vi "Drawing Tool.vi"() -> ()   [LabVIEW 2020]
doc: "An drawing tool that demonstrates the usage of LabVIEW object oriented programming"
uses:
  Picture/Picture.lvclass
  Graphics Object/Graphics Object.lvclass
  Color/Color.lvclass
  Line/Line.lvclass
  D:/Git/Labview-Libraries/Tools/Drawing Tool Folder/Graphics Object/Graphics Object.lvclass
  Rectangle/Rectangle.lvclass
  Circle/Circle.lvclass
  Triangle/Triangle.lvclass
  Ellipse/Ellipse.lvclass
  Empty/Empty.lvclass
  CMY Color/CMY Color.lvclass
  D:/Git/Labview-Libraries/Tools/Drawing Tool Folder/Color/Color.lvclass
  RGB Color/RGB Color.lvclass
  <vilib>/Utility/cursorutil.llb/Set Cursor (Icon Pict).vi
panel:
  in  "Undo":bool
  out "Colorbox":u32(colorbox)
  in  "Color":enum32{"RGB", "CMY"}(tab)
  in  "Blue RGB":u8(slide) caption="Blue" scale=0.0..255.0
  in  "Green RGB":u8(slide) caption="Green" scale=0.0..255.0
  in  "Red RGB":u8(slide) caption="Red" scale=0.0..255.0
  in  "Yellow CMY":u8(slide)=255 caption="Yellow" scale=0.0..255.0
  in  "Magenta CMY":u8(slide)=255 caption="Magenta" scale=0.0..255.0
  in  "Cyan CMY":u8(slide)=255 caption="Cyan" scale=0.0..255.0
  out "Tools":T1
  out "Picture":picture
  # "Color"
  # "expressionflow"
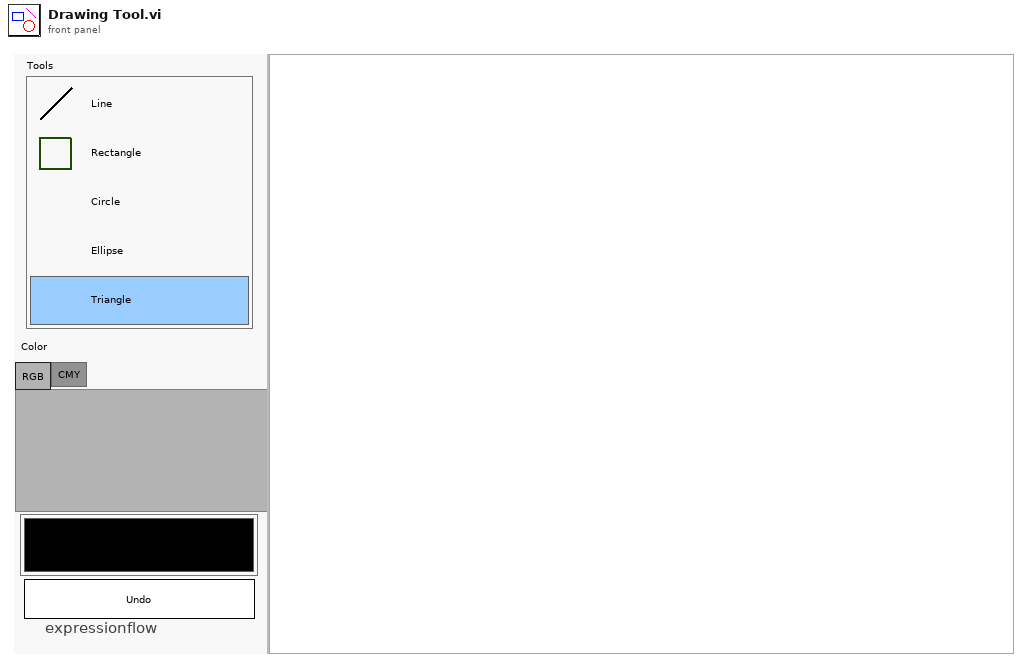
[diagram p1: front panel]
types:
  T1 = cluster{"Line":bool, "Rectangle":bool, "Circle":bool, "Ellipse":bool, "Triangle":bool}
  T2 = cluster{"Picture":refnum<class "Picture.lvclass">, "Tool":refnum<class "Graphics Object.lvclass">, "Unfinished Obj":refnum<class "Graphics Object.lvclass">, "Color":refnum<class "Color.lvclass">, "Tool":refnum<vi>, "Draw mode":bool}
  T3 = typedef "lveventtype.ctl" = enum32{"Null", "Timeout", "Annotation Menu Selection", "Annotation Menu Selection?", "App Instance Close", "App Instance Close?", "Autoscale Range Change", "Bookmark Info Change", "Cell Edit", "Cell Edit?", "Cursor Grab", "Cursor Grab?", "Cursor Menu Selection", "Cursor Menu Selection?", "Cursor Move", "Cursor Release", "Data Change", "Direction Change", "Display State Change", "Drag Ended", "Drag Enter", "Drag Leave", "Drag Over", "Drag Source Update", "Drag Starting", "Drag Starting?", "Drop", "Exec State Change", "Key Down", "Key Down?", "Key Repeat", "Key Repeat?", "Key Up", "Listbox Double Click", "Menu Activation?", "Menu Selection (App)", "Menu Selection? (App)", "Menu Selection (User)", "Mouse Down", "Mouse Down?", "Mouse Enter", "Mouse Leave", "Mouse Move", "Mouse Up", "Mouse Wheel", "NI Security User Change (App)", "Pane Size", "Panel Close", "Panel Close?", "Panel Resize", "Plot Attribute Change", "Scale Range Change", "Shortcut Menu Activation?", "Shortcut Menu Selection (App)", "Shortcut Menu Selection? (App)", "Shortcut Menu Selection (User)", "Tree Double Click", "Tree Drag", "Tree Drag?", "Tree Drop", "Tree Drop?", "Tree Item Close", "Tree Item Close?", "Tree Item Open", "Tree Item Open?", "User Event", "Value Change"}
  T4 = typedef "LVPoint32TypeDef.ctl" = cluster{"Horizontal":i32, "Vertical":i32}
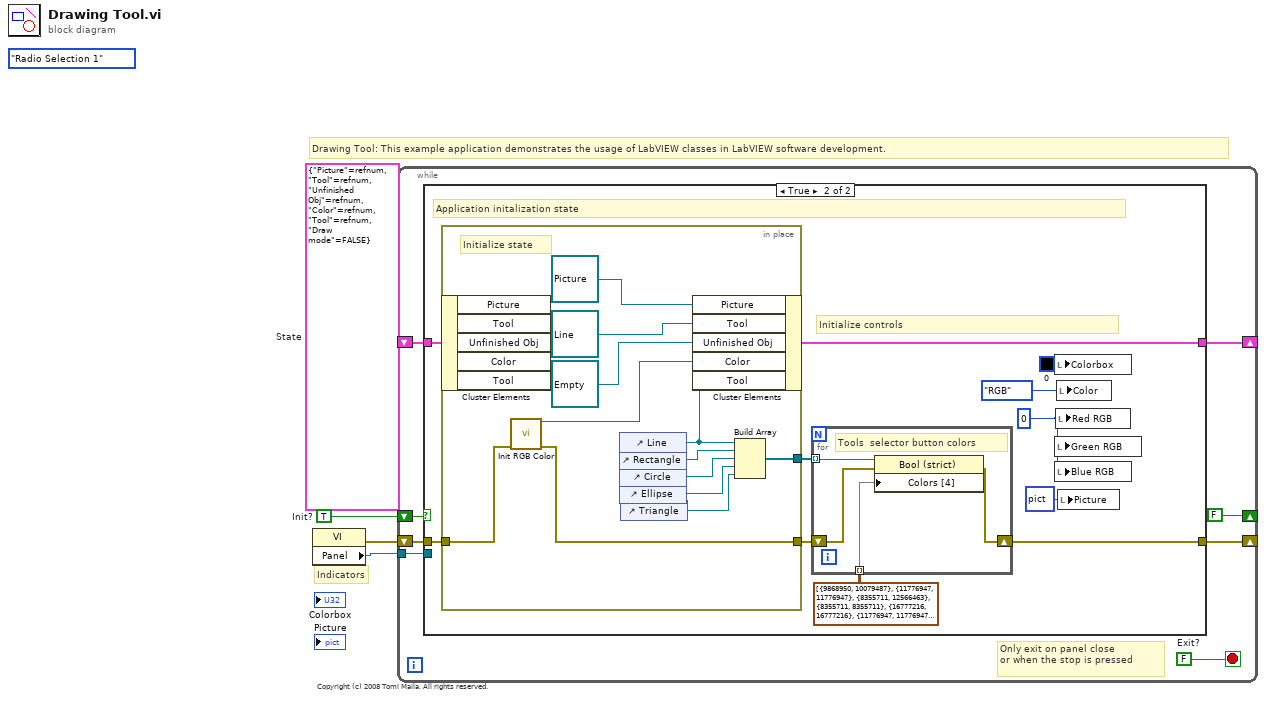
[diagram p0: block diagram]
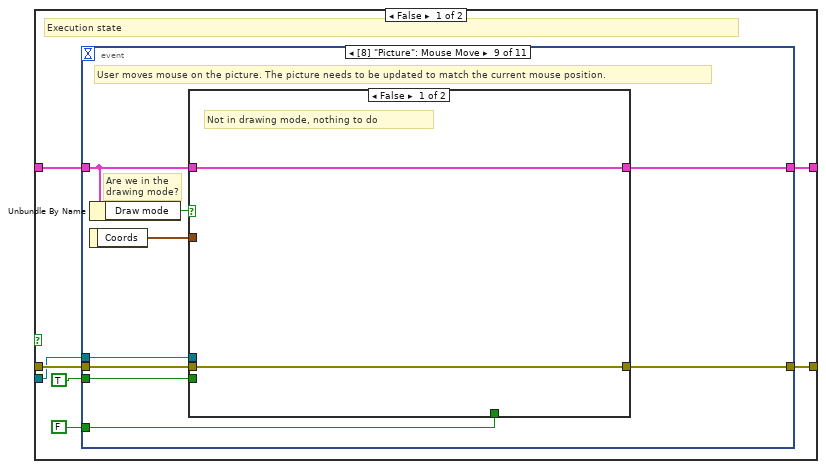
[diagram p2: hidden frame]
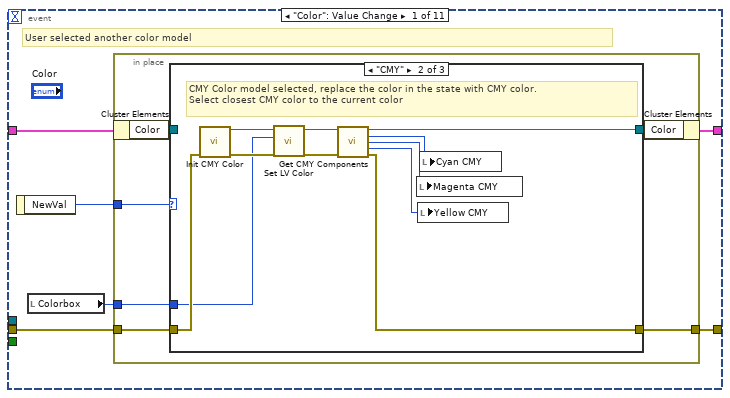
[diagram p3: hidden frame]
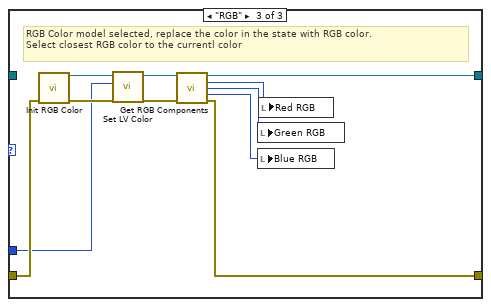
[diagram p5: hidden frame]
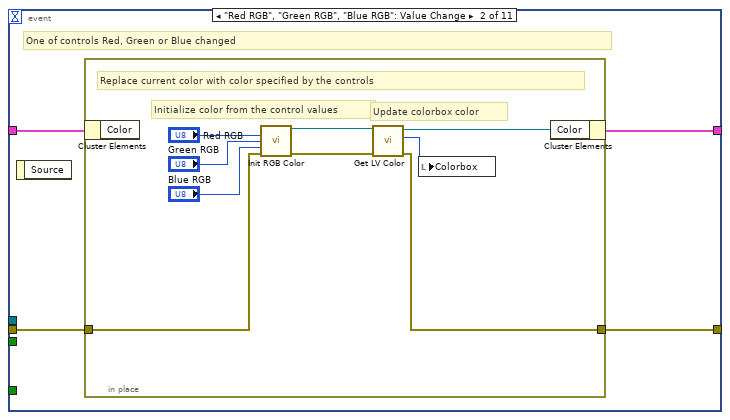
[diagram p6: hidden frame]
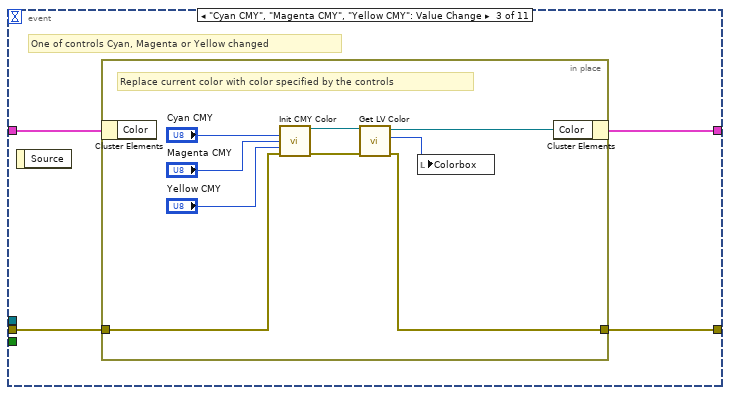
[diagram p7: hidden frame]
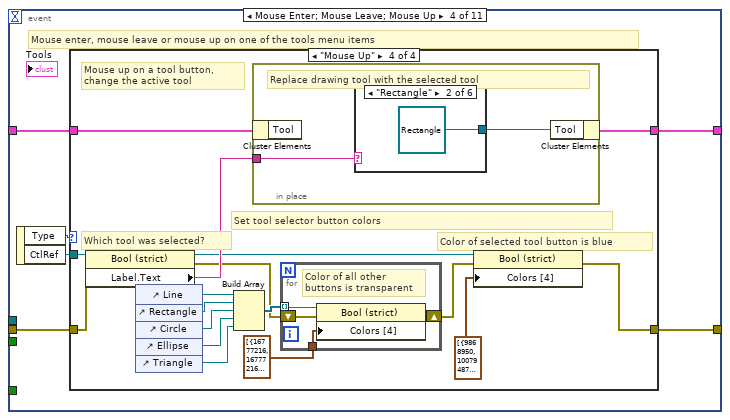
[diagram p8: hidden frame]
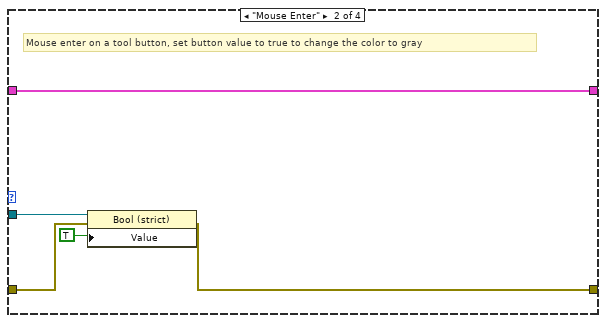
[diagram p10: hidden frame]
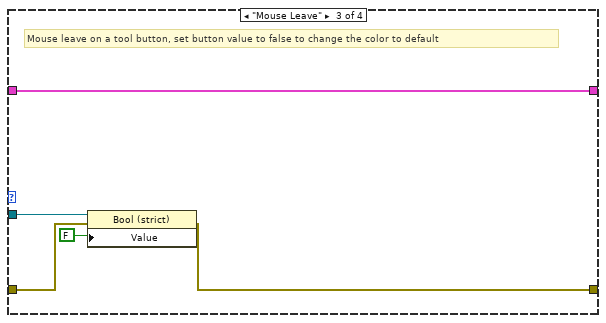
[diagram p11: hidden frame]
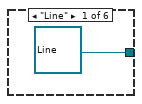
[diagram p12: hidden frame]
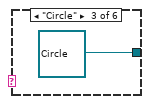
[diagram p13: hidden frame]
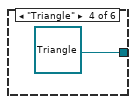
[diagram p14: hidden frame]
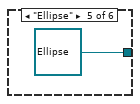
[diagram p15: hidden frame]
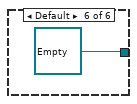
[diagram p16: hidden frame]
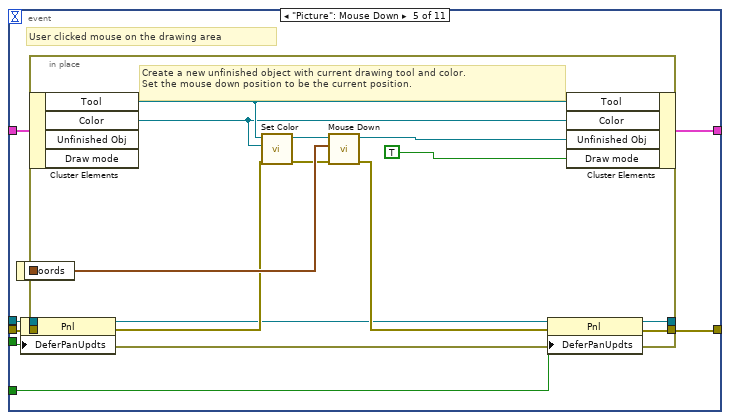
[diagram p17: hidden frame]
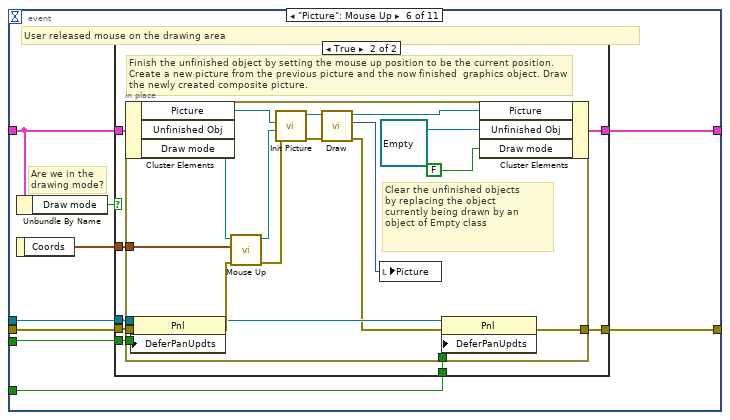
[diagram p18: hidden frame]
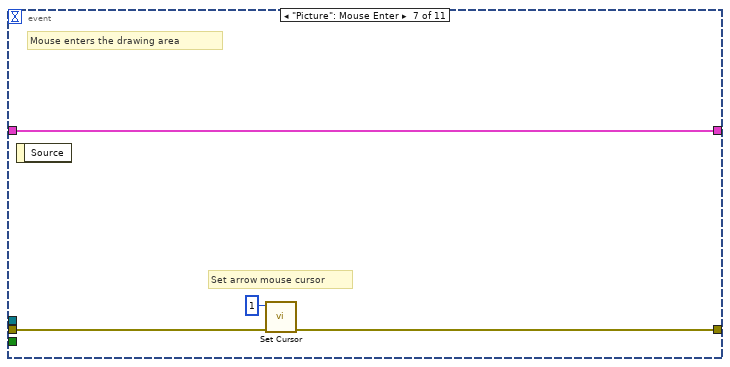
[diagram p20: hidden frame]
diagram:
  w1 = TRUE  # Init?
  w4 = T2 {"Picture"=refnum, "Tool"=refnum, "Unfinished Obj"=refnum, "Color"=refnum, "Tool"=refnum, "Draw mode"=FALSE}  # State
  (unwired) enum32{"Radio Selection 1", "Radio Selection 2"}."Radio Selection 1" ("Radio Buttons")
  # "Copyright (c) 2008 Tomi Maila. All rights reserved."
  # "Drawing Tool: This example application demonstrates the usage of LabVIEW classes in LabVIEW software development."
  # "Indicators"
  n1 = property class="VI"() -> (error out=w2:errorcluster, "Panel"=w3:refnum<vi>)  [unwired: 2 in, 1 out]
  n2 = while {
    shift-right: [w9] -> _
    shift-left: w2 -> [w10]
    shift-right: [w11] -> _
    shift-left: w4 -> [w12]
    tunnel: w3 -> [w7]
    shift-right: [FALSE ("Init?")] -> _
    shift-left: w1 -> [w8]
    stop <- w5 stop-if-true
    w5 = FALSE  # Exit?
    # "Only exit on panel close \nor when the stop is pressed"
    n3 = case shown="True" w8 {
      tunnel: w12 -> [w19 w274]
      tunnel: [w18 w272] -> w11
      tunnel: w10 -> [w17 w273]
      tunnel: w7 -> [w16 _]
      tunnel: [w13 w264] -> w9
      frame False {
        # "Execution state"
        n4 = event shown="[8] \"Picture\": Mouse Move" {
          selector: _ -> [_ _ _ _ _ _ _ _ _ _ _]
          dyn-events: _ -> [_ _ _ _ _ _ _ _ _ _ _]
          timeout: _ -> [_ _ _ _ _ _ _ _ _ _ _]
          tunnel: w17 -> [w25 w59 w72 w85 w134 w154 w191 w196 w205 w245 w259]
          tunnel: [w23 w58 w71 w84 w130 w152 w190 w195 w203 w241 w257] -> w13
          tunnel: w19 -> [w22 w57 w70 w83 w139 w157 w189 w194 w201 w248 w263]
          tunnel: [w21 w56 w69 w82 w138 w159 w189 w193 w207 w247 w263] -> w18
          tunnel: w16 -> [_ _ _ _ w137 w155 _ _ w206 w246 w258]
          tunnel: TRUE -> [_ _ _ _ w133 w153 _ _ w204 w244 _]
          tunnel: FALSE -> [_ _ _ _ w132 w151 _ _ w202 w239 _]
          event "Color": Value Change {
            # "User selected another color model"
            n5 = event-data() -> ("NewVal"=w24:enum32{"RGB", "CMY"})  [unwired: 1 in]
            n6 = local read "Colorbox"() -> (w20:u32)
            n7 = in-place {
              in-place-border: w20 -> [w31]
              in-place-border: w25 -> [w30]
              in-place-border: w24 -> [w29]
              in-place-border: [w26] -> w23
              n8 = in-place-cluster #1(w22) -> ("Color"=w27:refnum<class "Color.lvclass">)
              n9 = case shown="\"CMY\"" w29 {
                tunnel: w31 -> [_ w34 w45]
                tunnel: [w33 w42 w53] -> w28
                tunnel: [w32 w40 w51] -> w26
                tunnel: w30 -> [w32 w38 w49]
                tunnel: w27 -> [w33 _ _]
                frame Default {
                  # "Unknown color model"
                }
                frame "CMY" {
                  # "CMY Color model selected, replace the color in the state with CMY color.\nSelect closest CMY color to the current color"
                  n10 = call "Init CMY Color.vi"("error in (no error)"=w38) -> ("CMY Color out"=w44:refnum<class "CMY Color.lvclass">, "error out"=w39:errorcluster)  [unwired: 13 in]
                  n11 = call-dynamic "Set LV Color.vi"("error in (no error)"=w39, "Color (black)"=w34, "CMY Color.lvclass in"=w44) -> ("error out"=w41:errorcluster, "CMY Color.lvclass out"=w43:refnum<class "CMY Color.lvclass">)  [unwired: 7 in]
                  n12 = call-dynamic "Get CMY Components.vi"("CMY Color in"=w43, "error in (no error)"=w41) -> ("CMY Color out"=w42:refnum<class "CMY Color.lvclass">, "C"=w37:u8, "M"=w36:u8, "Y"=w35:u8, "error out"=w40:errorcluster)  [unwired: 9 in]
                  n13 = local write "Magenta CMY"(w36) -> ()
                  n14 = local write "Yellow CMY"(w35) -> ()
                  n15 = local write "Cyan CMY"(w37) -> ()
                }
                frame "RGB" {
                  # "RGB Color model selected, replace the color in the state with RGB color.\nSelect closest RGB color to the currentl color"
                  n16 = call "Init RGB Color.vi"("error in (no error)"=w49) -> ("RGB Color out"=w55:refnum<class "RGB Color.lvclass">, "error out"=w50:errorcluster)  [unwired: 13 in]
                  n17 = call-dynamic "Set LV Color.vi"("error in (no error)"=w50, "Color (black)"=w45, "RGB Color.lvclass in"=w55) -> ("error out"=w52:errorcluster, "RGB Color.lvclass out"=w54:refnum<class "RGB Color.lvclass">)  [unwired: 7 in]
                  n18 = call-dynamic "Get RGB Components.vi"("RGB Color in"=w54, "error in (no error)"=w52) -> ("RGB Color out"=w53:refnum<class "RGB Color.lvclass">, "R"=w48:u8, "G"=w47:u8, "B"=w46:u8, "error out"=w51:errorcluster)  [unwired: 9 in]
                  n19 = local write "Green RGB"(w47) -> ()
                  n20 = local write "Blue RGB"(w46) -> ()
                  n21 = local write "Red RGB"(w48) -> ()
                }
              }
              n22 = in-place-cluster #1("Color"=w28) -> (w21:T2)
            }
          }
          event "Red RGB", "Green RGB", "Blue RGB": Value Change {
            # "One of controls Red, Green or Blue changed"
            n23 = event-data() -> ()  [unwired: 1 in, 1 out]
            n24 = in-place {
              in-place-border: w59 -> [w66]
              in-place-border: [w64] -> w58
              # "Update colorbox color"
              # "Initialize color from the control values"
              # "Replace current color with color specified by the controls"
              n25 = in-place-cluster #2(w57) -> ()  [unwired: 1 out]
              n26 = call "Init RGB Color.vi"("R (0)"="Red RGB", "G (0)"="Green RGB", "B (0)"="Blue RGB", "error in (no error)"=w66) -> ("RGB Color out"=w68:refnum<class "RGB Color.lvclass">, "error out"=w67:errorcluster)  [unwired: 10 in]
              n27 = call-dynamic "Get LV Color.vi"("error in (no error)"=w67, "RGB Color.lvclass in"=w68) -> ("error out"=w64:errorcluster, "Color"=w63:u32, "RGB Color.lvclass out"=w65:refnum<class "RGB Color.lvclass">)  [unwired: 7 in]
              n28 = local write "Colorbox"(w63) -> ()
              n29 = in-place-cluster #2("Color"=w65) -> (w56:T2)
            }
          }
          event "Cyan CMY", "Magenta CMY", "Yellow CMY": Value Change {
            # "One of controls Cyan, Magenta or Yellow changed"
            n30 = event-data() -> ()  [unwired: 1 in, 1 out]
            n31 = in-place {
              in-place-border: w72 -> [w79]
              in-place-border: [w77] -> w71
              # "Replace current color with color specified by the controls"
              n32 = in-place-cluster #3(w70) -> ()  [unwired: 1 out]
              n33 = call "Init CMY Color.vi"("C (0)"="Cyan CMY", "M (0)"="Magenta CMY", "Y (0)"="Yellow CMY", "error in (no error)"=w79) -> ("CMY Color out"=w80:refnum<class "CMY Color.lvclass">, "error out"=w81:errorcluster)  [unwired: 10 in]
              n34 = call-dynamic "Get LV Color.vi"("error in (no error)"=w81, "CMY Color.lvclass in"=w80) -> ("error out"=w77:errorcluster, "Color"=w76:u32, "CMY Color.lvclass out"=w78:refnum<class "CMY Color.lvclass">)  [unwired: 7 in]
              n35 = local write "Colorbox"(w76) -> ()
              n36 = in-place-cluster #3("Color"=w78) -> (w69:T2)
            }
          }
          event "Tools.Line", "Tools.Rectangle", "Tools.Circle", "Tools.Ellipse", "Tools.Triangle": Mouse Enter; "Tools.Line", "Tools.Rectangle", "Tools.Circle", "Tools.Ellipse", "Tools.Triangle": Mouse Leave; "Tools.Line", "Tools.Rectangle", "Tools.Circle", "Tools.Ellipse", "Tools.Triangle": Mouse Up {
            # "Mouse enter, mouse leave or mouse up on one of the tools menu items"
            n37 = event-data() -> ("Type"=w87:T3, "CtlRef"=w86:refnum<vi>)  [unwired: 1 in]
            n38 = case shown="\"Mouse Up\"" w87 {
              tunnel: w86 -> [_ w94 w99 w116]
              tunnel: w85 -> [w89 w92 w97 w115]
              tunnel: [w89 w91 w96 w111] -> w84
              tunnel: w83 -> [w88 w90 w95 w114]
              tunnel: [w88 w90 w95 w113] -> w82
              frame Default {
                # "Unknown event, should never occur"
              }
              frame "Mouse Enter" {
                # "Mouse enter on a tool button, set button value to true to change the color to gray"
                n39 = property class="Bool (strict)"(reference=w94, error in=w92, "Value"=TRUE) -> (error out=w91:errorcluster)  [unwired: 1 out]
              }
              frame "Mouse Leave" {
                # "Mouse leave on a tool button, set button value to false to change the color to default"
                n40 = property class="Bool (strict)"(reference=w99, error in=w97, "Value"=FALSE) -> (error out=w96:errorcluster)  [unwired: 1 out]
              }
              frame "Mouse Up" {
                # "Mouse up on a tool button,\nchange the active tool"
                # "Which tool was selected?"
                # "Color of selected tool button is blue"
                # "Set tool selector button colors"
                n41 = property class="Bool (strict)"(reference=w116, error in=w115) -> (reference out=w101:refnum<vi>, error out=w103:errorcluster, "Label.Text"=w112:string)
                n42 = control-ref of="Line"() -> (w109:refnum<vi>)
                n43 = control-ref of="Rectangle"() -> (w108:refnum<vi>)
                n44 = control-ref of="Circle"() -> (w107:refnum<vi>)
                n45 = control-ref of="Ellipse"() -> (w106:refnum<vi>)
                n46 = control-ref of="Triangle"() -> (w100:refnum<vi>)
                n47 = Build Array(w109, w108, w107, w106, w100) -> (w104:refnum<vi>[])
                n48 = in-place {
                  in-place-border: w112 -> [w122]
                  # "Replace drawing tool with the selected tool"
                  n49 = in-place-cluster #4(w114) -> ()  [unwired: 1 out]
                  n50 = case shown="\"Rectangle\"" w122 {
                    tunnel: [refnum<class "Line.lvclass"> refnum ("Line.lvclass") refnum<class "Rectangle.lvclass"> refnum ("Rectangle.lvclass") refnum<class "Circle.lvclass"> refnum ("Circle.lvclass") refnum<class "Triangle.lvclass"> refnum ("Triangle.lvclass") refnum<class "Ellipse.lvclass"> refnum ("Ellipse.lvclass") refnum<class "Empty.lvclass"> refnum ("Empty.lvclass")] -> w121
                    frame "Line" {
                    }
                    frame "Rectangle" {
                    }
                    frame "Circle" {
                    }
                    frame "Triangle" {
                    }
                    frame "Ellipse" {
                    }
                    frame Default {
                    }
                  }
                  n51 = in-place-cluster #4("Tool"=w121) -> (w113:T2)
                }
                n52 = for {
                  shift-right: [w117] -> w102
                  shift-left: w103 -> [w119]
                  tunnel: w104 -> [w120] mode=indexing
                  tunnel: cluster{u32, u32}[] [{16777216, 16777216}, {11776947, 11776947}, {8355711, 12566463}, {8355711, 8355711}] ("Array 2") -> [w118]
                  # "Color of all other buttons is transparent"
                  n53 = property class="Bool (strict)"(reference=w120, error in=w119, "Colors [4]"=w118) -> (error out=w117:errorcluster)  [unwired: 1 out]
                }
                n54 = property class="Bool (strict)"(reference=w101, error in=w102, "Colors [4]"=cluster{u32, u32}[] [{9868950, 10079487}, {11776947, 11776947}, {8355711, 12566463}, {8355711, 8355711}] ("Array")) -> (error out=w111:errorcluster)  [unwired: 1 out]
              }
            }
          }
          event "Picture": Mouse Down {
            # "User clicked mouse on the drawing area"
            n55 = event-data() -> ("Coords"=w140:T4)  [unwired: 1 in]
            n56 = property class="Pnl"(reference=w137, error in=w134, "DeferPanUpdts"=w133) -> (reference out=w136:refnum<vi>, error out=w135:errorcluster)
            n57 = in-place {
              in-place-border: w140 -> [w149]
              in-place-border: [w150] -> w131
              in-place-border: w135 -> [w146]
              in-place-border: w136 -> [w144]
              in-place-border: [w144] -> w129
              # "Create a new unfinished object with current drawing tool and color. \nSet the mouse down position to be the current position."
              n58 = in-place-cluster #5(w139) -> ("Tool"=w147:refnum<class "Graphics Object.lvclass">, "Color"=w143:refnum<class "Color.lvclass">)  [unwired: 2 out]
              n59 = call-dynamic "Set Color.vi"("error in (no error)"=w146, "Color (RGB black)"=w143, "Geometric Object.lvclass in"=w147) -> ("error out"=w145:errorcluster, "Geometric Object.lvclass out"=w148:refnum<class "Graphics Object.lvclass">)  [unwired: 7 in]
              n60 = call-dynamic "Mouse Down.vi"("error in (no error)"=w145, "Point"=w149, "Geometric Object in"=w148) -> ("error out"=w150:errorcluster, "Geometric Object out"=w142:refnum<class "Graphics Object.lvclass">)  [unwired: 7 in]
              n61 = in-place-cluster #5("Tool"=w147, "Color"=w143, "Unfinished Obj"=w142, "Draw mode"=TRUE) -> (w138:T2)
            }
            n62 = property class="Pnl"(reference=w129, error in=w131, "DeferPanUpdts"=w132) -> (error out=w130:errorcluster)  [unwired: 1 out]
          }
          event "Picture": Mouse Up {
            # "Are we in the\ndrawing mode?"
            # "User released mouse on the drawing area"
            n63 = Unbundle By Name(w157) -> ("Draw mode"=w156:bool)
            n64 = event-data() -> ("Coords"=w158:T4)  [unwired: 1 in]
            n65 = case shown="True" w156 {
              tunnel: w157 -> [w161 w169]
              tunnel: [w161 w168] -> w159
              tunnel: w158 -> [_ w167]
              tunnel: w155 -> [_ w166]
              tunnel: w154 -> [w160 w165]
              tunnel: w153 -> [_ w164]
              tunnel: [w160 w163] -> w152
              tunnel: w151 -> [_ w162]
              frame False {
                # "Not in drawing mode"
              }
              frame True {
                # "Finish the unfinished object by setting the mouse up position to be the current position. Create a new picture from the previous picture and the now finished  graphics object. Draw the newly created composite picture."
                n66 = in-place {
                  in-place-border: w167 -> [w188]
                  in-place-border: w165 -> [w175]
                  in-place-border: w166 -> [w176]
                  in-place-border: w164 -> [w177]
                  in-place-border: [w171] -> w163
                  in-place-border: w162 -> [w170]
                  # "Clear the unfinished objects \nby replacing the object \ncurrently being drawn by an \nobject of Empty class"
                  n67 = in-place-cluster #6(w169) -> ("Picture"=w181:refnum<class "Picture.lvclass">, "Unfinished Obj"=w185:refnum<class "Graphics Object.lvclass">)  [unwired: 1 out]
                  n68 = property class="Pnl"(reference=w176, error in=w175, "DeferPanUpdts"=w177) -> (reference out=w173:refnum<vi>, error out=w174:errorcluster)
                  n69 = call-dynamic "Mouse Up.vi"("error in (no error)"=w174, "Point"=w188, "Geometric Object in"=w185) -> ("error out"=w183:errorcluster, "Geometric Object out"=w180:refnum<class "Graphics Object.lvclass">)  [unwired: 7 in]
                  n70 = call "Init Picture.vi"("error in (no error)"=w183, "New Object"=w180, "Previous Picture"=w181) -> ("error out"=w182:errorcluster, "Picture out"=w184:refnum<class "Picture.lvclass">)  [unwired: 7 in]
                  n71 = call-dynamic "Draw.vi"("error in (no error)"=w182, "Picture in"=w184) -> ("error out"=w172:errorcluster, "picture out"=w179:picture, "Picture out"=w187:refnum<class "Picture.lvclass">)  [unwired: 7 in]
                  n72 = local write "Picture"(w179) -> ()
                  n73 = property class="Pnl"(reference=w173, error in=w172, "DeferPanUpdts"=w170) -> (error out=w171:errorcluster)  [unwired: 1 out]
                  n74 = in-place-cluster #6("Picture"=w187, "Unfinished Obj"=refnum<class "Empty.lvclass"> refnum ("Tool"), "Draw mode"=FALSE) -> (w168:T2)
                }
              }
            }
          }
          event "Picture": Mouse Enter {
            # "Set arrow mouse cursor"
            # "Mouse enters the drawing area"
            n75 = event-data() -> ()  [unwired: 1 in, 1 out]
            n76 = call-poly <vilib>:"Set Cursor.vi"("error in (no error)"=w191, "icon"=u16 1) -> ("error out"=w190:errorcluster)  [unwired: 8 in, 1 out]
          }
          event "Picture": Mouse Leave {
            # "Set default mouose cursor"
            # "Mouse leaves the drawing area"
            n77 = event-data() -> ()  [unwired: 1 in, 1 out]
            n78 = in-place {
              # "Trun off the drawing mode"
              # "Clear the unfinished objects by replacing the object currently being drawn by an object of Empty class"
              n79 = in-place-cluster #7(w194) -> ()  [unwired: 2 out]
              n80 = in-place-cluster #7("Unfinished Obj"=refnum<class "Empty.lvclass"> refnum ("Tool"), "Draw mode"=FALSE) -> (w193:T2)
            }
            n81 = call-poly <vilib>:"Set Cursor.vi"("error in (no error)"=w196, "icon"=u16 0) -> ("error out"=w195:errorcluster)  [unwired: 8 in, 1 out]
          }
          event "Picture": Mouse Move {
            # "Are we in the\ndrawing mode?"
            # "User moves mouse on the picture. The picture needs to be updated to match the current mouse position."
            n82 = Unbundle By Name(w201) -> ("Draw mode"=w200:bool)
            n83 = event-data() -> ("Coords"=w208:T4)  [unwired: 1 in]
            n84 = case shown="False" w200 {
              tunnel: w208 -> [_ w218]
              tunnel: [w210 w217] -> w207
              tunnel: w206 -> [_ w216]
              tunnel: w205 -> [w209 w215]
              tunnel: w204 -> [_ w214]
              tunnel: [w209 w213] -> w203
              tunnel: w202 -> [_ w212]
              tunnel: w201 -> [w210 w211]
              frame False {
                # "Not in drawing mode, nothing to do"
              }
              frame True {
                # "Update the picture by drawing the current picture together with the\nunfinished picture with current mouse position."
                n85 = in-place {
                  in-place-border: w218 -> [w227]
                  in-place-border: w216 -> [w226]
                  in-place-border: w215 -> [w225]
                  in-place-border: w214 -> [w224]
                  in-place-border: [w220] -> w213
                  in-place-border: w212 -> [w219]
                  n86 = in-place-cluster #8(w211) -> ("Picture"=w231:refnum<class "Picture.lvclass">, "Unfinished Obj"=w229:refnum<class "Graphics Object.lvclass">)
                  n87 = property class="Pnl"(reference=w226, error in=w225, "DeferPanUpdts"=w224) -> (reference out=w222:refnum<vi>, error out=w223:errorcluster)
                  n88 = call-dynamic "Draw.vi"("error in (no error)"=w223, "Picture in"=w231) -> ("error out"=w232:errorcluster, "picture out"=w234:picture, "Picture out"=w230:refnum<class "Picture.lvclass">)  [unwired: 7 in]
                  n89 = call-dynamic "Mouse Move.vi"("error in (no error)"=w232, "Point"=w227, "Geometric Object in"=w229) -> ("error out"=w235:errorcluster, "Geometric Object out"=w233:refnum<class "Graphics Object.lvclass">)  [unwired: 7 in]
                  n90 = call-dynamic "Draw.vi"("error in (no error)"=w235, "picture in (empty picture)"=w234, "Geometric Object in"=w233) -> ("error out"=w221:errorcluster, "picture out"=w236:picture, "Geometric Object out"=w228:refnum<class "Graphics Object.lvclass">)  [unwired: 6 in]
                  n91 = local write "Picture"(w236) -> ()
                  n92 = in-place-cluster #8("Picture"=w230, "Unfinished Obj"=w228) -> (w217:T2)
                  n93 = property class="Pnl"(reference=w222, error in=w221, "DeferPanUpdts"=w219) -> (error out=w220:errorcluster)  [unwired: 1 out]
                }
              }
            }
          }
          event "Undo": Value Change {
            # "User pressed the undo button"
            n94 = event-data() -> ("NewVal"=w237:bool)  [unwired: 1 in]
            n95 = property class="Pnl"(reference=w246, error in=w245, "DeferPanUpdts"=w244) -> (reference out=w242:refnum<vi>, error out=w238:errorcluster)
            n96 = in-place {
              in-place-border: w238 -> [w251]
              in-place-border: [w256] -> w240
              in-place-border: [w253] -> w243
              in-place-border: w242 -> [w253]
              in-place-border: w237 -> [_]
              # "Request previous picture and draw it."
              n97 = in-place-cluster #9(w248) -> ("Picture"=w252:refnum<class "Picture.lvclass">)
              n98 = call "Undo.vi"("error in (no error)"=w251, "Picture.lvclass in"=w252) -> ("error out"=w249:errorcluster, "Picture.lvclass out"=w250:refnum<class "Picture.lvclass">)  [unwired: 7 in, 1 out]
              n99 = call-dynamic "Draw.vi"("error in (no error)"=w249, "Picture in"=w250) -> ("error out"=w256:errorcluster, "picture out"=w254:picture, "Picture out"=w255:refnum<class "Picture.lvclass">)  [unwired: 7 in]
              n100 = local write "Picture"(w254) -> ()
              n101 = in-place-cluster #9("Picture"=w255) -> (w247:T2)
            }
            n102 = property class="Pnl"(reference=w243, error in=w240, "DeferPanUpdts"=w239) -> (error out=w241:errorcluster)  [unwired: 1 out]
          }
          event Panel Close? {
            # "Show a dialog to verify exit."
            # "User wants to close the panel"
            n103 = event-data() -> ()  [unwired: 1 in, 1 out]
            n104 = Close Reference(reference=w258, error in (no error)=w259) -> (error out=w257:errorcluster)
            n105 = Two Button Dialog(message="Are you sure you want to exit the application?") -> (T button?=w262:bool)  [unwired: 2 in]
            n106 = Not(x=w262) -> (.not. x?=w261:bool)
            n107 = event-data("Discard?"=w261) -> ()  [unwired: 1 in, 1 out]
          }
        }
      }
      frame True {
        w270 = u8 0 ("Red RGB")
        # "Application initalization state"
        # "Initialize controls"
        n108 = in-place {
          in-place-border: w273 -> [w288]
          in-place-border: [w286] -> w267
          in-place-border: [w281] -> w266
          # "Initialize state"
          n109 = in-place-cluster #10(w274) -> ()  [unwired: 5 out]
          n110 = call "Init RGB Color.vi"("error in (no error)"=w288) -> ("RGB Color out"=w287:refnum<class "RGB Color.lvclass">, "error out"=w286:errorcluster)  [unwired: 13 in]
          n111 = control-ref of="Line"() -> (w280:refnum<vi>)
          n112 = control-ref of="Rectangle"() -> (w284:refnum<vi>)
          n113 = control-ref of="Circle"() -> (w283:refnum<vi>)
          n114 = control-ref of="Ellipse"() -> (w282:refnum<vi>)
          n115 = control-ref of="Triangle"() -> (w279:refnum<vi>)
          n116 = in-place-cluster #10("Picture"=refnum<class "Picture.lvclass"> refnum ("Picture.lvclass"), "Tool"=refnum<class "Line.lvclass"> refnum ("Line.lvclass"), "Unfinished Obj"=refnum<class "Empty.lvclass"> refnum ("Empty.lvclass"), "Color"=w287, "Tool"=w280) -> (w272:T2)
          n117 = Build Array(w280, w284, w283, w282, w279) -> (w281:refnum<vi>[])
        }
        n118 = for {
          shift-right: [w275] -> w264
          shift-left: w267 -> [w277]
          tunnel: w266 -> [w278] mode=indexing
          tunnel: cluster{u32, u32}[][] [[{9868950, 10079487}, {11776947, 11776947}, {8355711, 12566463}, {8355711, 8355711}], [{16777216, 16777216}, {11776947, 11776947}, {8355711, 12566463}, {8355711, 8355711}], [{16777216, 16777216}, {11776947, 11776947}, {8355711, 12566463}, {8355711, 8355711}], [{16777216, 16777216}, {11776947, 11776947}, {8355711, 12566463}, {8355711, 8355711}], [{16777216, 16777216}, {11776947, 11776947}, {8355711, 12566463}, {8355711, 8355711}]] ("Array 2") -> [w276] mode=indexing
          # "Tools  selector button colors"
          n119 = property class="Bool (strict)"(reference=w278, error in=w277, "Colors [4]"=w276) -> (error out=w275:errorcluster)  [unwired: 1 out]
        }
        n120 = local write "Colorbox"(u32 0 ("Colorbox")) -> ()
        n121 = local write "Green RGB"(w270) -> ()
        n122 = local write "Blue RGB"(w270) -> ()
        n123 = local write "Red RGB"(w270) -> ()
        n124 = local write "Color"(enum32{"RGB", "CMY"}."RGB" ("Color")) -> ()
        n125 = local write "Picture"(picture data[5B] ("Picture")) -> ()
      }
    }
  }
